vi "Last Ack.vi"(10 "Actor":refnum<class "Actor.lvclass">) -> (3 "Last Ack Msg out":refnum<class "Last Ack Msg.lvclass">)   [LabVIEW 2021, in "Last Ack.lvlib" / "Last Ack Msg.lvclass"]
uses:
  Last Ack Msg.lvclass
  Actor/Actor.lvclass
  Last Ack Msg.lvclass/Last Ack Msg.ctl
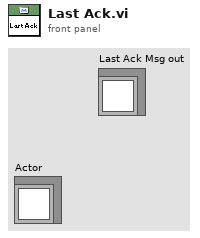
[diagram p1: front panel]
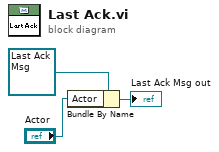
[diagram p0: block diagram]
diagram:
  n1 = Bundle By Name(cluster=refnum<class "Last Ack Msg.lvclass"> refnum ("Last Ack Msg in"), "Actor"="Actor") -> (→"Last Ack Msg out":refnum<class "Last Ack Msg.lvclass">)
